vi "tsdiag_can_create.vi"(10 "簇":T1, 11 "路径输入":path) -> (2 "返回类型":i32, 3 "路径输出":path)   [LabVIEW 2019]
panel:
  out "pDiagModuleIndex":i32
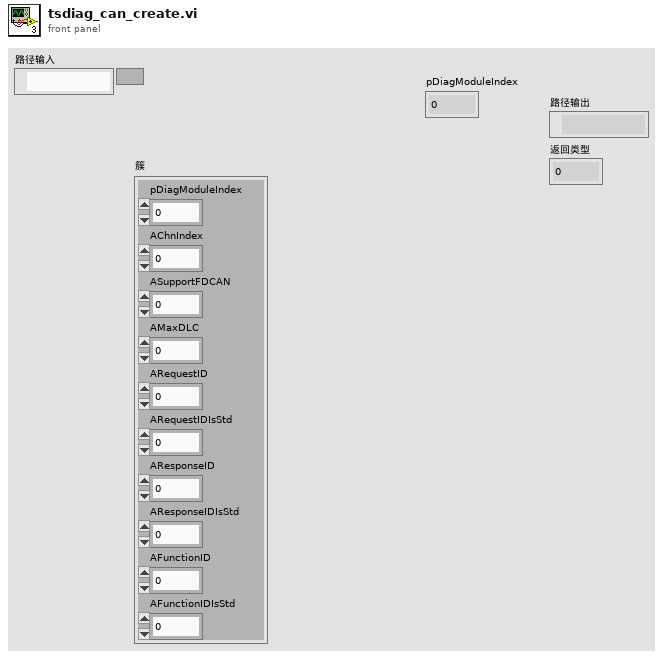
[diagram p1: front panel]
types:
  T1 = cluster{"pDiagModuleIndex":i32, "AChnIndex":i32, "ASupportFDCAN":i16, "AMaxDLC":u8, "ARequestID":u32, "ARequestIDIsStd":i32, "AResponseID":u32, "AResponseIDIsStd":i32, "AFunctionID":u32, "AFunctionIDIsStd":u8}
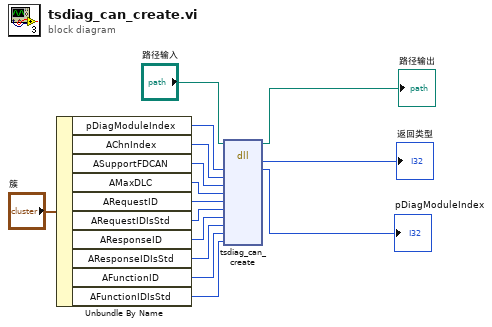
[diagram p0: block diagram]
diagram:
  n1 = Unbundle By Name("簇") -> ("pDiagModuleIndex"=w11:i32, "AChnIndex"=w10:i32, "ASupportFDCAN"=w9:i16, "AMaxDLC"=w8:u8, "ARequestID"=w7:u32, "ARequestIDIsStd"=w6:i32, "AResponseID"=w5:u32, "AResponseIDIsStd"=w4:i32, "AFunctionID"=w3:u32, "AFunctionIDIsStd"=w2:u8)
  n2 = dll-call lib="C:/Users/XYY/Desktop/LabView Demo/TSCAN_LB2018_V1.3_20220301/Config/TSMaster.dll" fn="tsdiag_can_create"(path in="路径输入", "pDiagModuleIndex"=w11, "AChnIndex"=w10, "ASupportFDCAN"=w9, "AMaxDLC"=w8, "ARequestID"=w7, "ARequestIDIsStd"=w6, "AResponseID"=w5, "AResponseIDIsStd"=w4, "AFunctionID"=w3, "AFunctionIDIsStd"=w2) -> (path out=→"路径输出":path, "返回类型"=→"返回类型":i32, "pDiagModuleIndex"=→"pDiagModuleIndex":i32)  [unwired: 11 in, 1 out]
